vi "Close Device Core.vi"(8 "error in (no error)":errorcluster, 11 "CS++Nanotec in":refnum<class "CS++Nanotec.lvclass">) -> (0 "error out":errorcluster, 3 "CS++Nanotec out":refnum<class "CS++Nanotec.lvclass">)   [LabVIEW 2015, in "CS++Nanotec.lvlib" / "CS++Nanotec.lvclass"]
doc: "Close device driver connection."
uses:
  CS++Nanotec.lvclass
  CS++Nanotec.lvclass/CS++Nanotec.ctl
  CSPP_DeviceBase/CS++Motor/CS++Motor.lvclass
  instr.lib/NanotecSMCPD/NanotecSMCPDDriver.lvlib
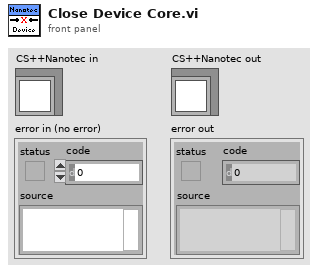
[diagram p1: front panel]
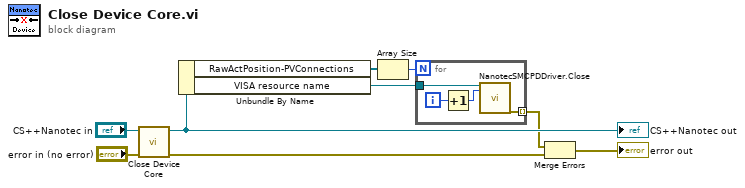
[diagram p0: block diagram]
diagram:
  n1 = call-parent "Close Device Core.vi"("error in (no error)"="error in (no error)", "CS++Motor in"="CS++Nanotec in") -> ("error out"=w3:errorcluster, "CS++Motor out"=w7:refnum<class "CS++Nanotec.lvclass">)  [unwired: 8 in]
  "CS++Nanotec out" <- w7
  n2 = Unbundle By Name(w7) -> ("RawActPosition-PVConnections"=w5:refnum<class "PVConnection.lvclass">[], "VISA resource name"=w6:refnum<visa-resource-name>)
  n3 = Array Size(array=w5) -> (size(s)=w4:i32)
  n4 = for {
    N: w4 -> [_]
    tunnel: w6 -> [w13]
    tunnel: [w10] -> w1 mode=indexing
    i -> [w11]
    n5 = Increment(x=w11) -> (x+1=w12:i32)
    n6 = call "NanotecSMCPDDriver.Close.vi"("VISA resource name"=w13, "contollerID"=w12) -> ("error out"=w10:errorcluster)  [unwired: 17 in]
  }
  n7 = Merge Errors(w1, w3) -> (→"error out":errorcluster)
